vi "NUMBER_FROM_STRING_ARRAY.vi"(11 "Table List":string[](array[string])) -> (3 "Array":string[](array[string]))   [LabVIEW 2017]
uses:
  <vilib>/regexp/Match Regular Expression.xnode
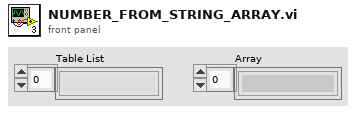
[diagram p1: front panel]
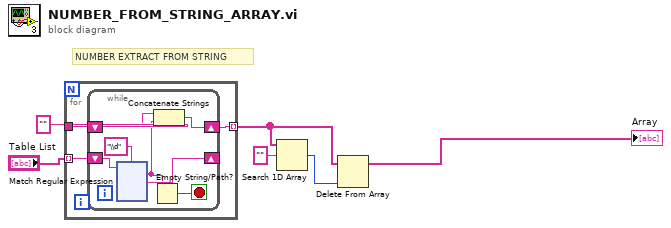
[diagram p0: block diagram]
diagram:
  # "NUMBER EXTRACT FROM STRING"
  n1 = for {
    tunnel: [w9] -> w3 mode=indexing
    tunnel: "" -> [w8]
    tunnel: "Table List" -> [w7] mode=indexing
    n2 = while {
      shift-right: [w13] -> _
      shift-left: w7 -> [w16]
      shift-right: [w11] -> w9
      shift-left: w8 -> [w12]
      stop <- w14 stop-if-true
      n3 = xnode "Match Regular Expression"("input string"=w16, "regular expression"="\\d") -> ("whole match"=w10:string, "after match"=w13:string)  [unwired: 4 in, 3 out]
      n4 = Empty String/Path?(string/path=w10) -> (empty?=w14:bool)
      n5 = Concatenate Strings(w12, w10) -> (w11:string)
    }
  }
  n6 = Search 1D Array(1D array=w3, element="") -> (index of element=w1:i32)  [unwired: 1 in]
  n7 = Delete From Array(array=w3, index=w1) -> (array with subset deleted=→"Array":string[])  [unwired: 1 in, 1 out]
